vi "DT_Triangle Manager_Add.vi"(9 "Triangle":i32[](array[numeric]), 10 "next triangle in":i32, 11 "Triangles In":i32[][](array[numeric])) -> (2 "next triangle out":i32, 3 "Triangles Out":i32[][](array[numeric]))   [LabVIEW 2020, in "NI_AAL_Geometry.lvlib"]
uses:
  <vilib>/Analysis/NI_AAL_Geometry.lvlib
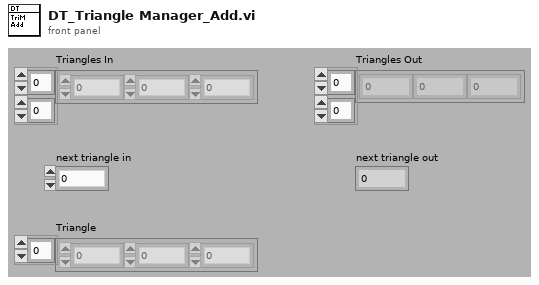
[diagram p1: front panel]
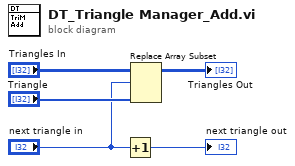
[diagram p0: block diagram]
diagram:
  n1 = Increment(x="next triangle in") -> (x+1=→"next triangle out":i32)
  n2 = Replace Array Subset(array="Triangles In", new element="Triangle", index (row)="next triangle in") -> (→"Triangles Out":i32[][])  [unwired: 1 in]
